vi "ThresholdBurst.vi"(2 "# bins":i32, 3 "Array":dbl[](array[numeric]) format="%.2f") -> (0 "Best Fit Coefficients":dbl[](array[numeric]) format="%.2f", 1 "Intensity-Histogram":cluster{"Axis":dbl[], "Histogram":i32[]}(graph))   [LabVIEW 2009]
uses:
  <vilib>/Analysis/NI_AALPro.lvlib
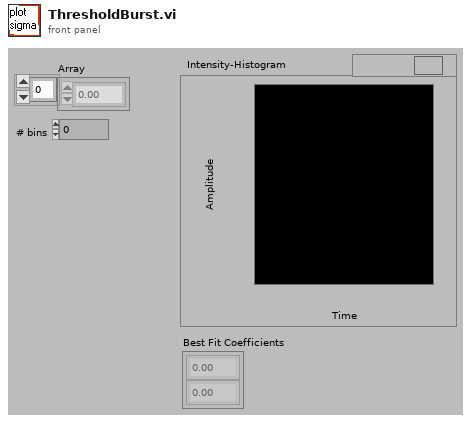
[diagram p1: front panel]
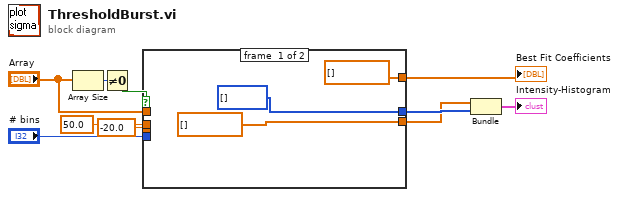
[diagram p0: block diagram]
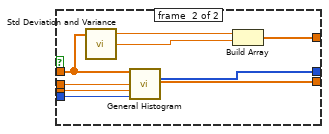
[diagram p2: hidden frame]
diagram:
  n1 = Array Size(array="Array") -> (size(s)=w10:i32)
  n2 = Not Equal To 0?(x=w10) -> (x != 0?=w9:bool)
  n3 = case shown="True" w9 {
    tunnel: "Array" -> [_ w17]
    tunnel: [i32[] [] ("Histogram") w22] -> w4
    tunnel: [dbl[] [] ("Axis") w21] -> w3
    tunnel: -20.0 ("min") -> [_ w20]
    tunnel: 50.0 ("max") -> [_ w19]
    tunnel: "# bins" -> [_ w18]
    tunnel: [dbl[] [] w15] -> w2
    frame #0 {
    }
    frame #1 {
      n4 = call "Std Deviation and Variance.vi"("X"=w17) -> ("mean"=w16:dbl, "standard deviation"=w14:dbl)  [unwired: 1 in, 1 out]
      n5 = call <vilib>:"General Histogram.vi"("X"=w17, "max"=w19, "min"=w20, "# bins"=w18) -> ("Histogram"=w22:i32[], "Axis"=w21:dbl[])  [unwired: 7 in, 3 out]
      n6 = Build Array(w16, w14) -> (w15:dbl[])
    }
  }
  "Best Fit Coefficients" <- w2
  n7 = Bundle("Axis"=w3, "Histogram"=w4) -> (→"Intensity-Histogram":cluster{"Axis":dbl[], "Histogram":i32[]})  [unwired: 1 in]
